vi "save data to disk.vi"(0 "disk queues":T2, 1 "refnums":T1, 5 "error in":errorcluster) -> (14 "files open":bool, 19 "error out":errorcluster)   [LabVIEW 2017]
uses:
  typedefs/queue cluster.ctl
  typedefs/reading queue.ctl
  typedefs/reading.ctl
  typedefs/readingType.ctl
  typedefs/reading1.ctl
  typedefs/refnum cluster.ctl
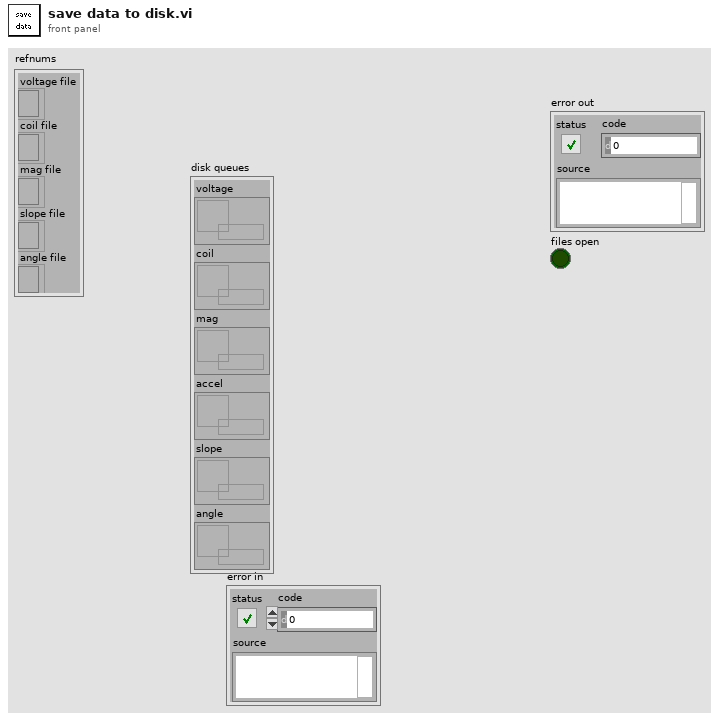
[diagram p1: front panel]
types:
  T1 = typedef "refnum cluster.ctl" = cluster{"voltage file":refnum<file>, "coil file":refnum<file>, "mag file":refnum<file>, "slope file":refnum<file>, "angle file":refnum<file>}
  T2 = typedef "queue cluster.ctl" = cluster{"voltage":T3, "coil":T3, "mag":T3, "accel":T3, "slope":refnum<queue>, "angle":refnum<queue>}
  T3 = typedef "reading queue.ctl" = refnum<queue>
  T4 = typedef "reading.ctl" = cluster{"reading type":T5, "time":fxp<+,48,48>, "x":sgl, "y":sgl, "z":sgl, "XSUM":u8}
  T5 = typedef "readingType.ctl" = enum8{"SYNC", "DETVAL", "COILI", "MAGVEC", "ACCVEC"}
  T6 = typedef "reading1.ctl" = cluster{"time":dbl, "x":dbl, "ms timer":u32}
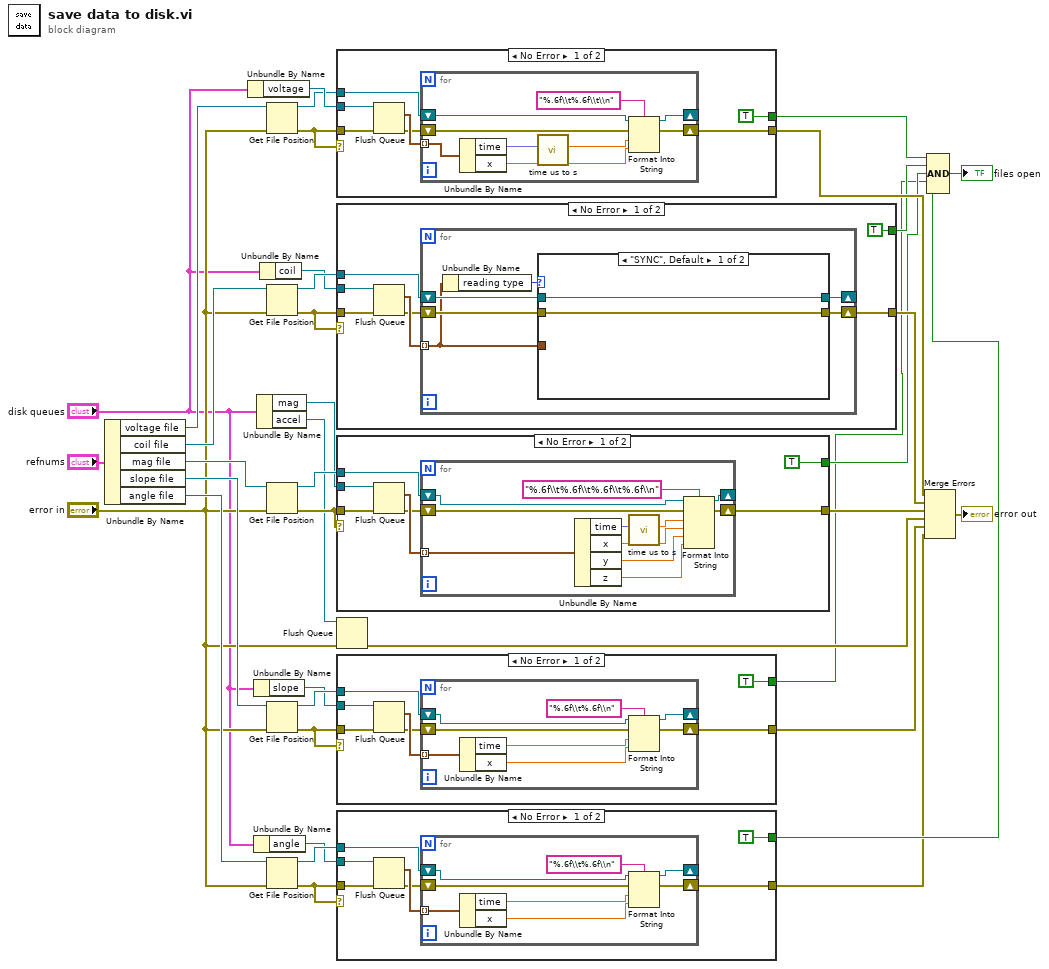
[diagram p0: block diagram]
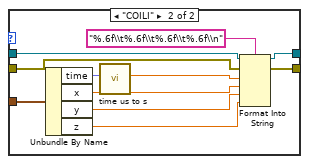
[diagram p5: hidden frame]
diagram:
  n1 = Unbundle By Name("refnums") -> ("voltage file"=w19:refnum<file>, "coil file"=w20:refnum<file>, "mag file"=w21:refnum<file>, "slope file"=w8:refnum<file>, "angle file"=w7:refnum<file>)
  n2 = Unbundle By Name("disk queues") -> ("voltage"=w37:T3)
  n3 = Unbundle By Name("disk queues") -> ("slope"=w12:refnum<queue>)
  n4 = Unbundle By Name("disk queues") -> ("angle"=w9:refnum<queue>)
  n5 = Unbundle By Name("disk queues") -> ("mag"=w29:T3, "accel"=w28:T3)
  n6 = Unbundle By Name("disk queues") -> ("coil"=w32:T3)
  n7 = Get File Position(4:"error in", 7:w19) -> (0:w35:errorcluster, 3:w36:refnum<file>)  [unwired: 1 out]
  n8 = Get File Position(4:"error in", 7:w20) -> (0:w33:errorcluster, 3:w34:refnum<file>)  [unwired: 1 out]
  n9 = Get File Position(4:"error in", 7:w21) -> (0:w30:errorcluster, 3:w31:refnum<file>)  [unwired: 1 out]
  n10 = Get File Position(4:"error in", 7:w8) -> (0:w13:errorcluster, 3:w14:refnum<file>)  [unwired: 1 out]
  n11 = Get File Position(4:"error in", 7:w7) -> (0:w10:errorcluster, 3:w11:refnum<file>)  [unwired: 1 out]
  n12 = case shown="No Error" w35 {
    tunnel: w37 -> [w44 _]
    tunnel: w35 -> [w41 _]
    tunnel: w36 -> [w40 _]
    tunnel: [w39 _] -> w24
    tunnel: [TRUE _] -> w16
    frame No Error {
      n13 = Flush Queue(queue=w44, error in (no error)=w41) -> (remaining elements=w43:T4[], error out=w42:errorcluster)  [unwired: 1 out]
      n14 = for {
        tunnel: w43 -> [w52] mode=indexing
        shift-right: [w48] -> _
        shift-left: w40 -> [w47]
        shift-right: [w46] -> w39
        shift-left: w42 -> [w49]
        n15 = Unbundle By Name(w52) -> ("time"=w51:fxp<+,48,48>, "x"=w50:sgl)
        n16 = call "time us to s.vi"("time (us)"=w51) -> ("time (s)"=w45:dbl)  [unwired: 10 in]
        n17 = Format Into String(format string="%.6f\\t%.6f\\t\\n", initial string=w47, error in=w49, w45, w50) -> (resulting string=w48:refnum<file>, error out=w46:errorcluster)
      }
    }
    frame Error {
    }
  }
  n18 = case shown="No Error" w33 {
    tunnel: w32 -> [w60 _]
    tunnel: w33 -> [w57 _]
    tunnel: w34 -> [w56 _]
    tunnel: [w55 _] -> w25
    tunnel: [TRUE _] -> w17
    frame No Error {
      n19 = Flush Queue(queue=w60, error in (no error)=w57) -> (remaining elements=w59:T4[], error out=w58:errorcluster)  [unwired: 1 out]
      n20 = for {
        tunnel: w59 -> [w62] mode=indexing
        shift-right: [w65] -> _
        shift-left: w56 -> [w64]
        shift-right: [w63] -> w55
        shift-left: w58 -> [w66]
        n21 = Unbundle By Name(w62) -> ("reading type"=w61:T5)
        n22 = case shown="\"SYNC\", Default" w61 {
          tunnel: w62 -> [_ w79]
          tunnel: w66 -> [w67 w77]
          tunnel: [w68 w76] -> w65
          tunnel: w64 -> [w68 w75]
          tunnel: [w67 w74] -> w63
          frame "SYNC", Default {
          }
          frame "COILI" {
            n23 = Unbundle By Name(w79) -> ("time"=w73:fxp<+,48,48>, "x"=w78:sgl, "y"=w70:sgl, "z"=w69:sgl)
            n24 = call "time us to s.vi"("time (us)"=w73) -> ("time (s)"=w72:dbl)  [unwired: 10 in]
            n25 = Format Into String(format string="%.6f\\t%.6f\\t%.6f\\t%.6f\\n", initial string=w75, error in=w77, w72, w78, w70, w69) -> (resulting string=w76:refnum<file>, error out=w74:errorcluster)
          }
        }
      }
    }
    frame Error {
    }
  }
  n26 = case shown="No Error" w30 {
    tunnel: w29 -> [w86 _]
    tunnel: w30 -> [w83 _]
    tunnel: w31 -> [w82 _]
    tunnel: [w81 _] -> w26
    tunnel: [TRUE _] -> w18
    frame No Error {
      n27 = Flush Queue(queue=w86, error in (no error)=w83) -> (remaining elements=w85:T4[], error out=w84:errorcluster)  [unwired: 1 out]
      n28 = for {
        tunnel: w85 -> [w96] mode=indexing
        shift-right: [w92] -> _
        shift-left: w82 -> [w91]
        shift-right: [w90] -> w81
        shift-left: w84 -> [w93]
        n29 = Unbundle By Name(w96) -> ("time"=w88:fxp<+,48,48>, "x"=w95:sgl, "y"=w94:sgl, "z"=w89:sgl)
        n30 = call "time us to s.vi"("time (us)"=w88) -> ("time (s)"=w87:dbl)  [unwired: 10 in]
        n31 = Format Into String(format string="%.6f\\t%.6f\\t%.6f\\t%.6f\\n", initial string=w91, error in=w93, w87, w95, w94, w89) -> (resulting string=w92:refnum<file>, error out=w90:errorcluster)
      }
    }
    frame Error {
    }
  }
  n32 = Flush Queue(queue=w28, error in (no error)="error in") -> (error out=w27:errorcluster)  [unwired: 2 out]
  n33 = case shown="No Error" w13 {
    tunnel: w12 -> [w104 _]
    tunnel: w13 -> [w101 _]
    tunnel: w14 -> [w100 _]
    tunnel: [w99 _] -> w2
    tunnel: [TRUE _] -> w4
    frame No Error {
      n34 = Flush Queue(queue=w104, error in (no error)=w101) -> (remaining elements=w103:T6[], error out=w102:errorcluster)  [unwired: 1 out]
      n35 = for {
        tunnel: w103 -> [w111] mode=indexing
        shift-right: [w107] -> _
        shift-left: w100 -> [w106]
        shift-right: [w105] -> w99
        shift-left: w102 -> [w108]
        n36 = Unbundle By Name(w111) -> ("time"=w110:dbl, "x"=w109:dbl)
        n37 = Format Into String(format string="%.6f\\t%.6f\\n", initial string=w106, error in=w108, w110, w109) -> (resulting string=w107:refnum<file>, error out=w105:errorcluster)
      }
    }
    frame Error {
    }
  }
  n38 = case shown="No Error" w10 {
    tunnel: w9 -> [w119 _]
    tunnel: w10 -> [w116 _]
    tunnel: w11 -> [w115 _]
    tunnel: [w114 _] -> w1
    tunnel: [TRUE _] -> w3
    frame No Error {
      n39 = Flush Queue(queue=w119, error in (no error)=w116) -> (remaining elements=w118:T6[], error out=w117:errorcluster)  [unwired: 1 out]
      n40 = for {
        tunnel: w118 -> [w126] mode=indexing
        shift-right: [w122] -> _
        shift-left: w115 -> [w121]
        shift-right: [w120] -> w114
        shift-left: w117 -> [w123]
        n41 = Unbundle By Name(w126) -> ("time"=w125:dbl, "x"=w124:dbl)
        n42 = Format Into String(format string="%.6f\\t%.6f\\n", initial string=w121, error in=w123, w125, w124) -> (resulting string=w122:refnum<file>, error out=w120:errorcluster)
      }
    }
    frame Error {
    }
  }
  n43 = Merge Errors(w24, w25, w26, w27, w2, w1) -> (→"error out":errorcluster)
  n44 = Compound Arithmetic op=AND(w16, w17, w18, w4, w3) -> (→"files open":bool)
